vi "FSM.vi"() -> ()   [LabVIEW 2022 SP3]
panel:
  in  "generator on/off":bool
  out "Waveform Chart":dbl(graph)
  out "State off - first, on -second":bool
  in  "state controller off - first state, on - second state":bool
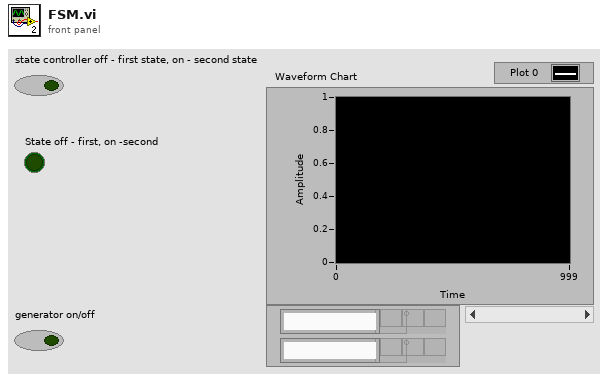
[diagram p1: front panel]
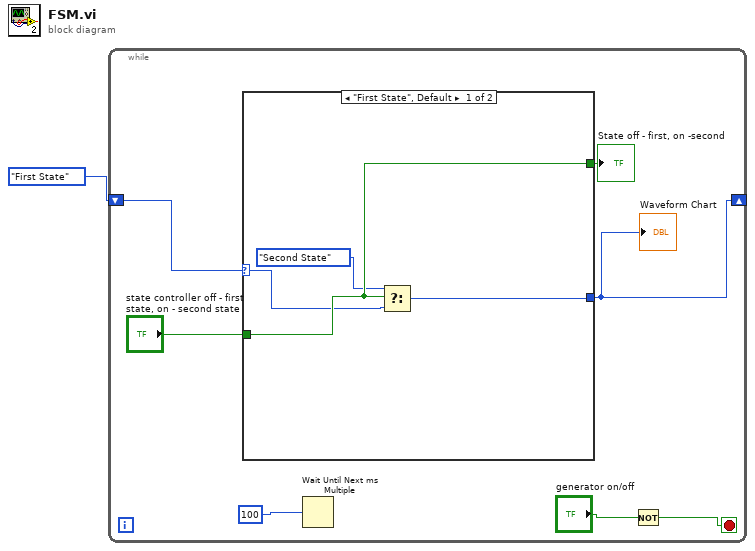
[diagram p0: block diagram]
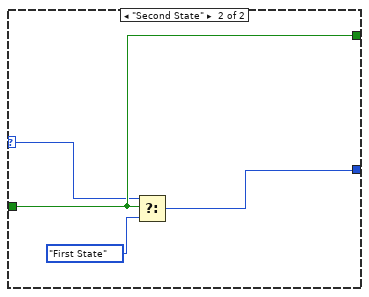
[diagram p2: hidden frame]
diagram:
  n1 = while {
    shift-right: [w2] -> _
    shift-left: enum16{"First State", "Second State", ""}."First State" -> [w8]
    stop <- w3 stop-if-true
    n2 = case shown="\"First State\", Default" w8 {
      selector: w8 -> [w9 w13]
      tunnel: "state controller off - first state, on - second state" -> [w12 w15]
      tunnel: [w12 w15] -> w6
      tunnel: [w11 w14] -> w2
      frame "First State", Default {
        n3 = Select(t=enum16{"First State", "Second State", ""}."Second State", s=w12, f=w9) -> (s? t:f=w11:enum16{"First State", "Second State", ""})
      }
      frame "Second State" {
        n4 = Select(t=w13, s=w15, f=enum16{"First State", "Second State", ""}."First State") -> (s? t:f=w14:enum16{"First State", "Second State", ""})
      }
    }
    "State off - first, on -second" <- w6
    "Waveform Chart" <- w2
    n5 = Wait Until Next ms Multiple(millisecond multiple=100) -> ()  [unwired: 1 out]
    n6 = Not(x="generator on/off") -> (.not. x?=w3:bool)
  }
